vi "Reduce Funds and Check.vi"(8 "error in (no error)":errorcluster, 10 "Amount to Reduce":u32, 11 "Data Cluster":T1) -> (0 "error out":errorcluster, 1 "Remaining Balance":u32, 2 "Sucessful":bool, 3 "Data Cluster Out":T1)   [LabVIEW 2019, in "Money.lvlib"]
uses:
  Money.lvlib
  Module Data--cluster.ctl
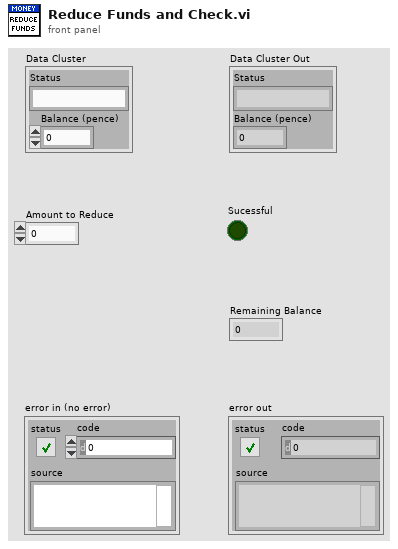
[diagram p1: front panel]
types:
  T1 = typedef "Money.lvlib/Module Data--cluster.ctl" = cluster{"Status":string, "Balance (pence)":u32}
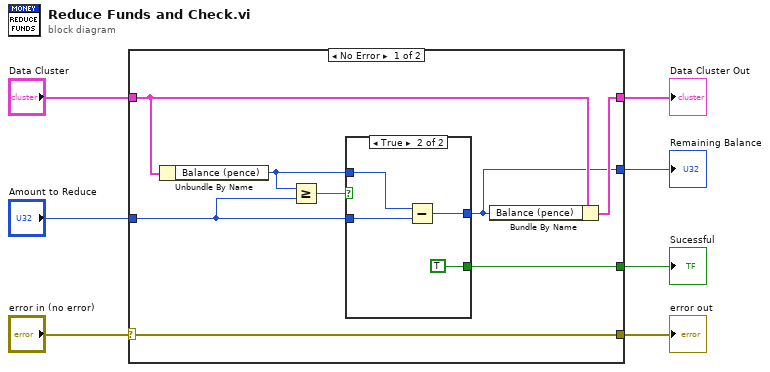
[diagram p0: block diagram]
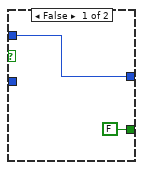
[diagram p2: hidden frame]
diagram:
  n1 = case shown="No Error" "error in (no error)" {
    selector: "error in (no error)" -> [w15 w23]
    tunnel: "Data Cluster" -> [w13 w22]
    tunnel: [w12 w22] -> w6
    tunnel: [w15 w23] -> w4
    tunnel: "Amount to Reduce" -> [w9 _]
    tunnel: [w14 _] -> w2
    tunnel: [w8 _] -> w1
    frame No Error {
      n2 = Unbundle By Name(w13) -> ("Balance (pence)"=w11:u32)
      n3 = Greater Or Equal?(x=w11, y=w9) -> (x >= y?=w10:bool)
      n4 = case shown="True" w10 {
        tunnel: [FALSE TRUE] -> w14
        tunnel: [w17 w18] -> w8
        tunnel: w11 -> [w17 w20]
        tunnel: w9 -> [_ w19]
        frame False {
        }
        frame True {
          n5 = Subtract(x=w20, y=w19) -> (x-y=w18:u32)
        }
      }
      n6 = Bundle By Name(cluster=w13, "Balance (pence)"=w8) -> (w12:T1)
    }
    frame Error {
    }
  }
  "Data Cluster Out" <- w6
  "error out" <- w4
  "Sucessful" <- w2
  "Remaining Balance" <- w1
